vi "gvbooleschRT.vi"() -> ()   [LabVIEW 2017]
panel:
  in  "global stop RT":bool
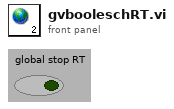
[diagram p1: front panel]
diagram:
